vi "analysis tester.vi"() -> ()   [LabVIEW 2020]
uses:
  Image analysys result.ctl
panel:
  out "Image Analysis Result":T1 {"MaxCounts" format="%.2p"; "FWHMy" format="%.2p"; "FWHMx" format="%.2p"; "MeanCounts" format="%.2p"; "CentroidY" format="%.2p"; "CentroidX" format="%.2p"}
  out "Image Out 2":T2(plugin-control)
  out "Image Out":T2(plugin-control)
  in  "File Path":path
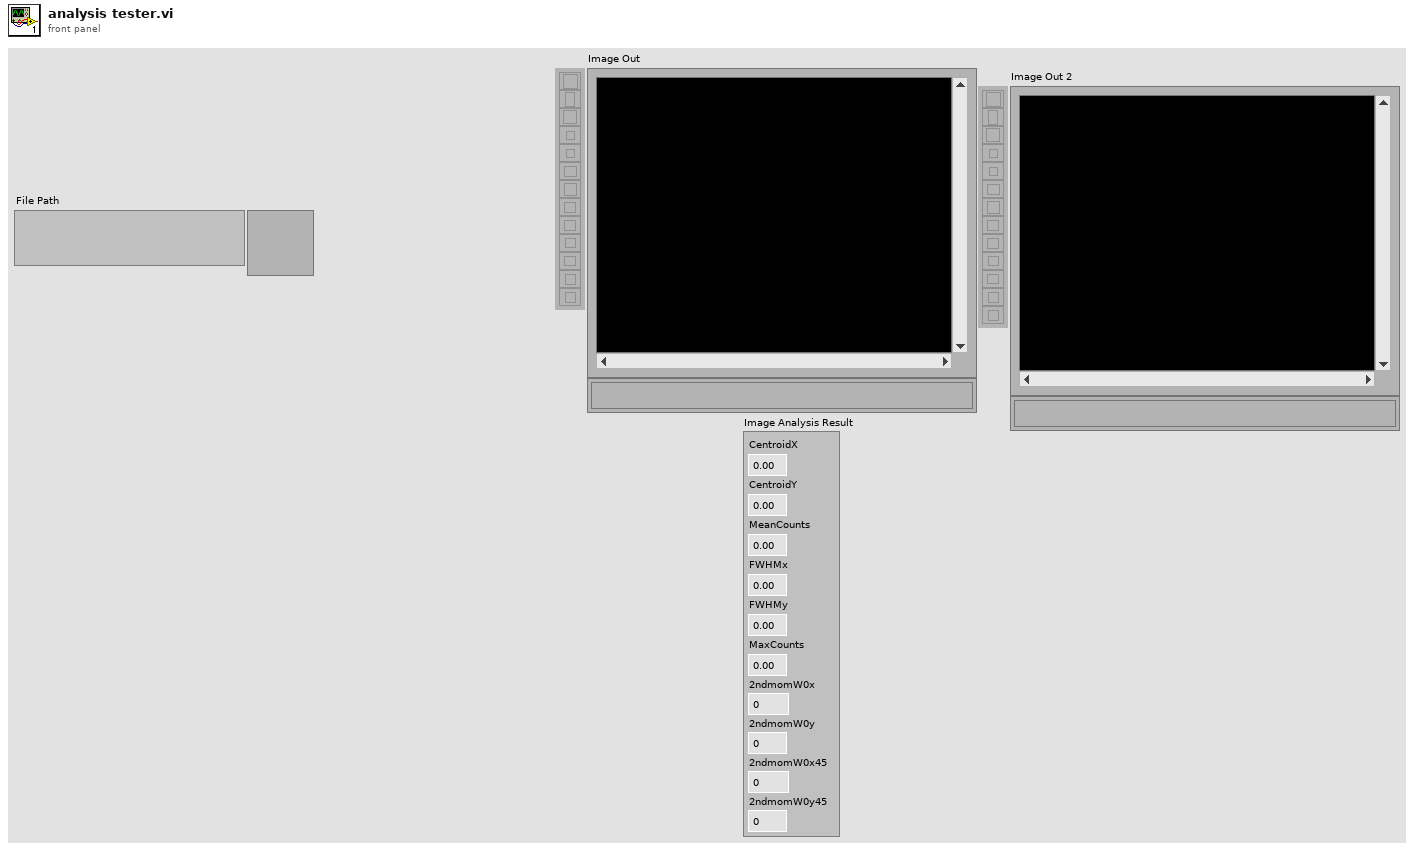
[diagram p1: front panel]
types:
  T1 = typedef "Image analysys result.ctl" = cluster{"CentroidX":sgl, "CentroidY":sgl, "MeanCounts":sgl, "FWHMx":sgl, "FWHMy":sgl, "MaxCounts":sgl, "2ndmomW0x":sgl, "2ndmomW0y":sgl, "2ndmomW0x45":sgl, "2ndmomW0y45":sgl}
  T2 = typedef "IMAQ Image.ctl" = refnum<image>
  T3 = typedef "Image Type" = u32
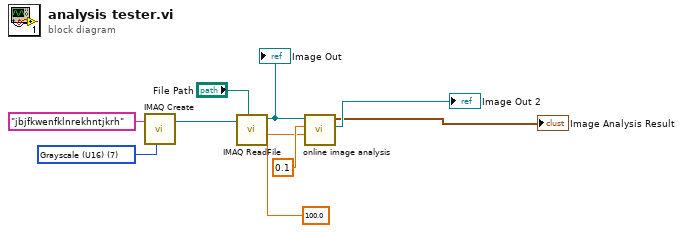
[diagram p0: block diagram]
diagram:
  w7 = T3 7 items=["Grayscale (U8)", "Grayscale (I16)", "Grayscale (SGL)", "Complex (CSG)", "RGB (U32)", "HSL (U32)", "RGB (U64)", "Grayscale (U16)"] ("Image Type")
  n1 = call "IMAQ Create"("Image Name"="jbjfkwenfklnrekhntjkrh", "Image Type"=w7) -> ("New Image"=w6:T2)  [unwired: 3 in, 1 out]
  n2 = call "IMAQ ReadFile"("File Path"="File Path", "Image"=w6) -> ("Image Out"=w9:T2)  [unwired: 5 in, 4 out]
  "Image Out" <- w9
  n3 = call "online image analysis.vi"("half width for 2nd mom cut"=sgl 100.0, "Threshold"=0.1, "Refnum in"=w9) -> ("Image"=→"Image Out 2":T2, "Image Analysis Result"=→"Image Analysis Result":T1)  [unwired: 6 in, 1 out]
